vi "Get_MultiVar_Value.vi"(8 "error in (no error)":errorcluster, 10 "varName":string, 11 "mupExpr in":refnum<data-value>) -> (0 "error out":errorcluster, 2 "Value":dbl, 3 "mupExpr out":refnum<data-value>)   [LabVIEW 2015, in "mupExpr.lvclass"]
uses:
  mupExpr.lvclass
  mupExpr.lvclass/mupExpr.ctl
  <vilib>/Utility/error.llb/Error Cluster From Error Code.vi
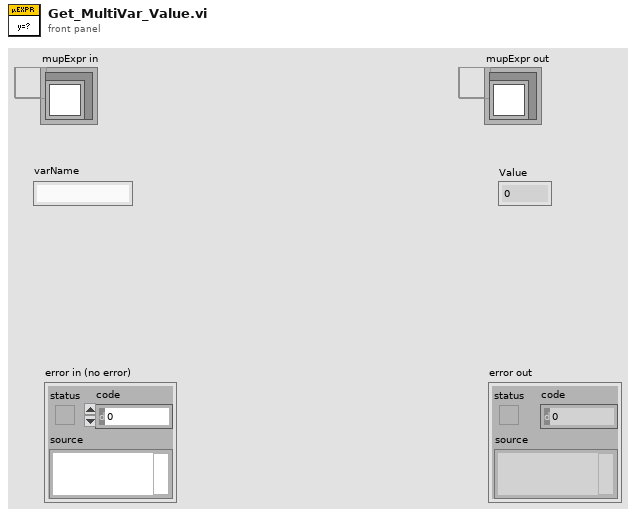
[diagram p1: front panel]
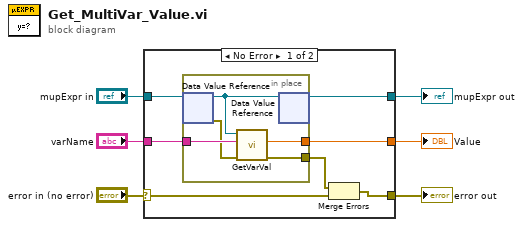
[diagram p0: block diagram]
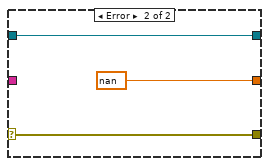
[diagram p2: hidden frame]
diagram:
  n1 = case shown="No Error" "error in (no error)" {
    selector: "error in (no error)" -> [w10 w21]
    tunnel: [w8 w21] -> w5
    tunnel: [w11 w20] -> w3
    tunnel: "mupExpr in" -> [w12 w20]
    tunnel: [w13 nan ("pd")] -> w2
    tunnel: "varName" -> [w7 _]
    frame No Error {
      n2 = in-place {
        in-place-border: [w15] -> w9
        in-place-border: [w16] -> w13
        in-place-border: w7 -> [w18]
        n3 = in-place-dvr #1(w12) -> (w17:refnum<class "mupExpr.lvclass">, w14:errorcluster)
        n4 = call "GetVarVal.vi"("error in (no error)"=w14, "varName"=w18, "muExpr in"=w17) -> ("error out"=w15:errorcluster, "varValue"=w16:dbl)  [unwired: 6 in, 1 out]
        n5 = in-place-dvr #1(w17) -> (w11:refnum<data-value>)  [unwired: 1 out]
      }
      n6 = Merge Errors(w9, w10) -> (w8:errorcluster)
    }
    frame Error {
    }
  }
  "error out" <- w5
  "mupExpr out" <- w3
  "Value" <- w2
